vi "write.vi"(6 "FilePath":refnum<vi>, 7 "Rec Flag Reference":refnum<vi>, 8 "error in (no error)":errorcluster, 9 "Save Flag Reference":refnum<vi>, 10 "Stop Flag Reference":refnum<vi>, 11 "Photodiode in":refnum<class "Photodiode.lvclass">) -> (0 "error out":errorcluster, 3 "Photodiode out":refnum<class "Photodiode.lvclass">)   [LabVIEW 2016, in "Photodiode.lvclass"]
uses:
  Photodiode.lvclass
  Photodiode.lvclass/Photodiode.ctl
  private/HDF5Tools32/LabView/Append To Dataset 2D Double.vi
  private/HDF5Tools32/LabView/HDF5Tools.lvlib
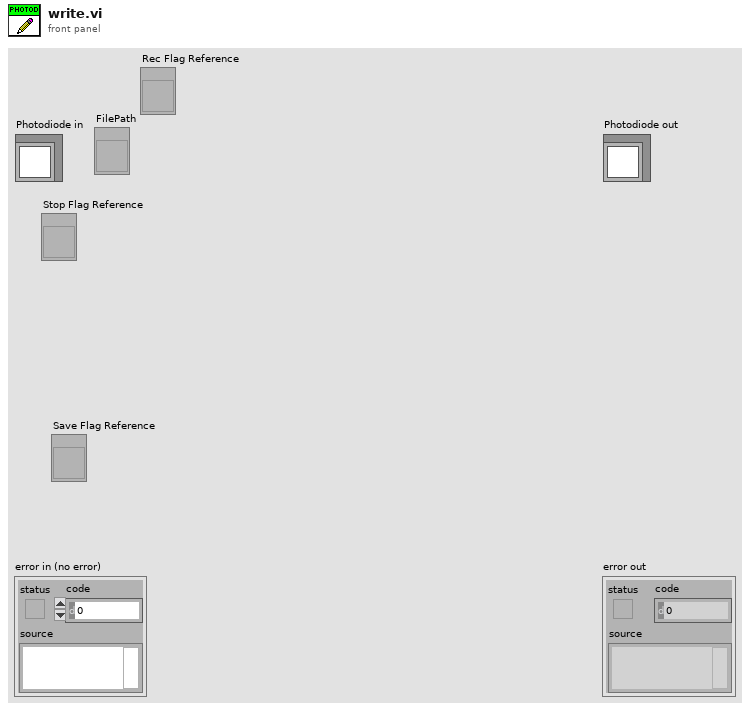
[diagram p1: front panel]
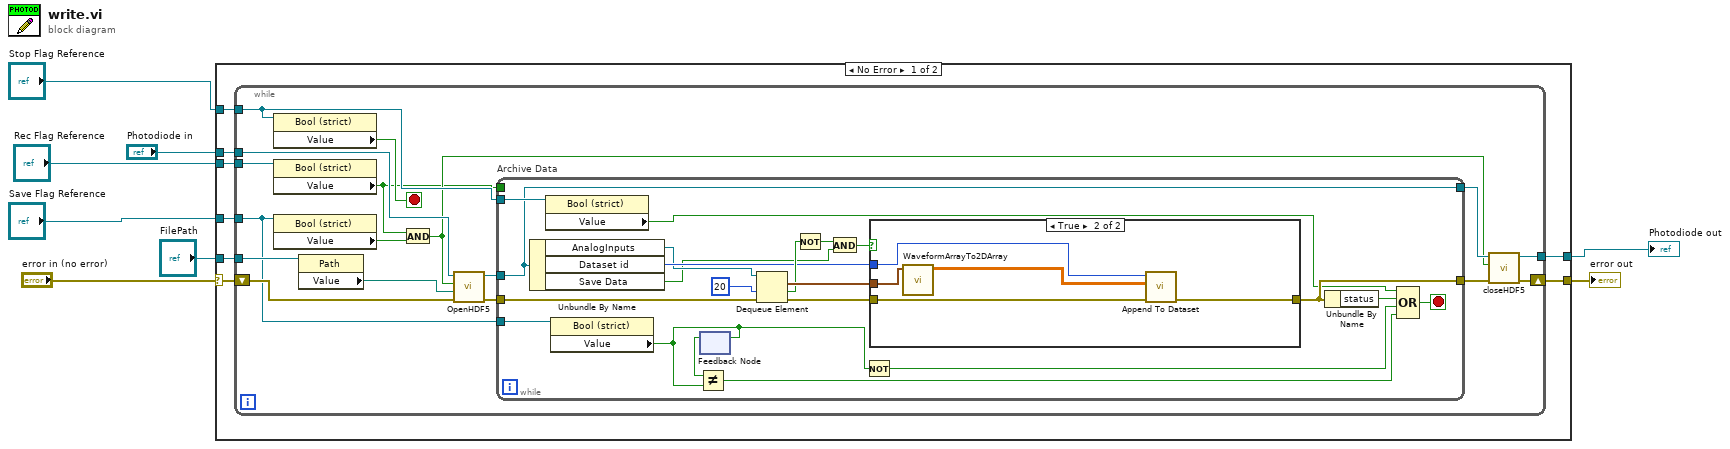
[diagram p0: block diagram]
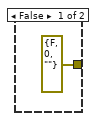
[diagram p2: hidden frame]
diagram:
  n1 = case shown="No Error" "error in (no error)" {
    selector: "error in (no error)" -> [w15 w62]
    tunnel: [w16 w62] -> w7
    tunnel: [w12 w61] -> w5
    tunnel: "Photodiode in" -> [w13 w61]
    tunnel: "Stop Flag Reference" -> [w14 _]
    tunnel: "Save Flag Reference" -> [w11 _]
    tunnel: "FilePath" -> [w10 _]
    tunnel: "Rec Flag Reference" -> [w9 _]
    frame No Error {
      n2 = while {
        tunnel: w14 -> [w25]
        tunnel: w13 -> [w33]
        shift-right: [w27] -> w16
        shift-left: w15 -> [w30]
        tunnel: [w26] -> w12
        tunnel: w11 -> [w22]
        tunnel: w10 -> [w24]
        tunnel: w9 -> [w17]
        stop <- w19 stop-if-true
        n3 = property class="Bool (strict)"(reference=w25) -> ("Value"=w19:bool)  [unwired: 1 in, 2 out]
        n4 = property class="Bool (strict)"(reference=w17) -> ("Value"=w18:bool)  [unwired: 1 in, 2 out]
        n5 = property class="Bool (strict)"(reference=w22) -> ("Value"=w21:bool)  [unwired: 1 in, 2 out]
        n6 = property class="Path"(reference=w24) -> ("Value"=w23:path)  [unwired: 1 in, 2 out]
        n7 = And(x=w18, y=w21) -> (x .and. y?=w20:bool)
        n8 = call-dynamic "OpenHDF5.vi"("error in (no error)"=w30, "appended path"=w23, "Save Analog Signals"=w20, "Photodiode in"=w33) -> ("error out"=w29:errorcluster, "Photodiode out"=w32:refnum<class "Photodiode.lvclass">)  [unwired: 6 in]
        n9 = while "Archive Data" {
          tunnel: [w51] -> w28
          tunnel: w29 -> [w49]
          tunnel: w25 -> [w48]
          tunnel: w32 -> [w45]
          tunnel: [w45] -> w31
          tunnel: w18 -> [_]
          tunnel: w22 -> [w41]
          stop <- w42 stop-if-true
          n10 = Unbundle By Name(w45) -> ("AnalogInputs"=w46:refnum<queue>, "Dataset id"=w47:i32, "Save Data"=w34:bool)
          n11 = property class="Bool (strict)"(reference=w48) -> ("Value"=w44:bool)  [unwired: 1 in, 2 out]
          n12 = property class="Bool (strict)"(reference=w41) -> ("Value"=w38:bool)  [unwired: 1 in, 2 out]
          n13 = feedback #1() -> (w40:bool)  [unwired: 1 in]
          n14 = Not Equal?(x=w40, y=w38) -> (x != y?=w37:bool)
          n15 = feedback-in #1(w38) -> ()
          n16 = Dequeue Element(queue=w46, timeout in ms (-1)=20, error in (no error)=w49) -> (element=w53:waveform(dbl)[], timed out?=w50:bool, error out=w52:errorcluster)  [unwired: 1 out]
          n17 = Not(x=w50) -> (.not. x?=w35:bool)
          n18 = And(x=w35, y=w34) -> (x .and. y?=w36:bool)
          n19 = Not(x=w38) -> (.not. x?=w39:bool)
          n20 = case shown="True" w36 {
            tunnel: w53 -> [_ w60]
            tunnel: [errorcluster {"status"=FALSE, "code"=0, "source"=""} ("Error out") w58] -> w51
            tunnel: w52 -> [_ w57]
            tunnel: w47 -> [_ w56]
            frame False {
            }
            frame True {
              n21 = call "WaveformArrayTo2DArray.vi"("Waveform Array"=w60) -> ("2-D Array"=w59:dbl[][])  [unwired: 10 in]
              n22 = call-poly "Append To Dataset.vi"("Error in (no error)"=w57, "Data"=w59, "Dataset id in"=w56) -> ("Error out"=w58:errorcluster)  [unwired: 7 in, 1 out]
            }
          }
          n23 = Unbundle By Name(w51) -> ("status"=w43:bool)
          n24 = Compound Arithmetic op=OR(w44, w43, w39, w37) -> (w42:bool)
        }
        n25 = call-dynamic "closeHDF5.vi"("error in (no error)"=w28, "Save Analog Signals"=w20, "Photodiode in"=w31) -> ("error out"=w27:errorcluster, "Photodiode out"=w26:refnum<class "Photodiode.lvclass">)  [unwired: 7 in]
      }
    }
    frame Error {
    }
  }
  "error out" <- w7
  "Photodiode out" <- w5
